vi "Format Epoch Time.vi"(8 "UTC? (F)":bool, 9 "Fractional Second":dbl format="%#.6f", 10 "System Time (s)":i64, 11 "DateTimeFormatter in":refnum<class "DateTimeFormatter.lvclass">) -> (0 "Not a Timestamp?":bool, 2 "DateTime String":string, 3 "DateTimeFormatter out":refnum<class "DateTimeFormatter.lvclass">)   [LabVIEW 2013, in "DateTimeFormatter.lvclass"]
uses:
  DateTimeFormatter.lvclass
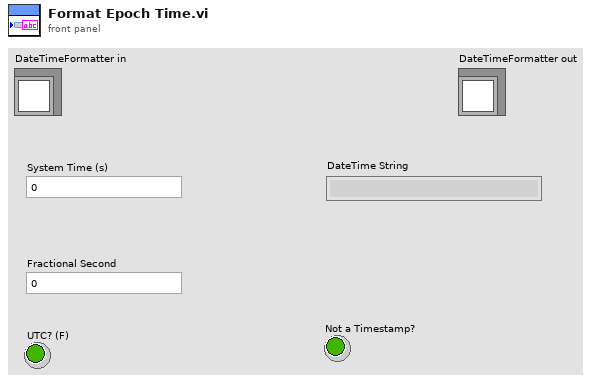
[diagram p1: front panel]
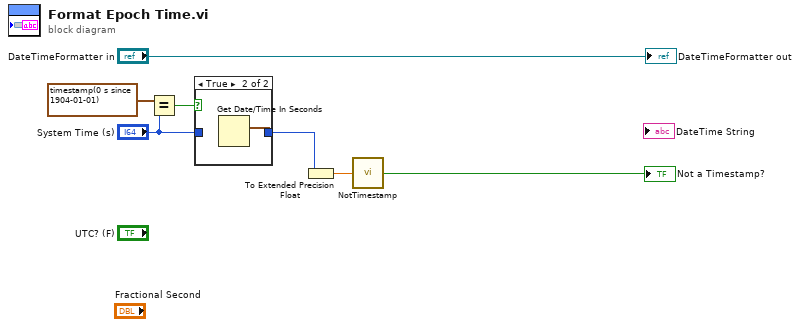
[diagram p0: block diagram]
diagram:
  n1 = Equal?(x=timestamp(0 s since 1904-01-01), y="System Time (s)") -> (x = y?=w5:bool)
  n2 = case shown="True" w5 {
    tunnel: [w8 w9] -> w3
    tunnel: "System Time (s)" -> [w8 _]
    frame False {
    }
    frame True {
      n3 = Get Date/Time In Seconds() -> (seconds since 1Jan1904=w9:timestamp)
    }
  }
  n4 = To Extended Precision Float(1:w3) -> (0:w2:ext)
  n5 = call "NotTimestamp.vi"("value"=w2) -> ("Not a Timestamp?"=→"Not a Timestamp?":bool)  [unwired: 4 in]
  "DateTimeFormatter out" <- "DateTimeFormatter in"
